vi "读取AVI文件V0（简化版）.vi"() -> ()   [LabVIEW 2013]
panel:
  in  "延时":u32
  in  "value":bool
  in  "AVI File Path":path
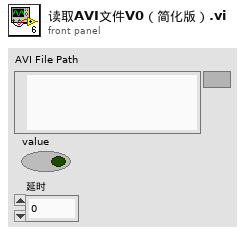
[diagram p1: front panel]
types:
  T1 = typedef "IMAQ AVI2 Refnum.ctl" = refnum<k20>
  T2 = typedef "Image Type" = u32
  T3 = typedef "IMAQ Image.ctl" = refnum<image>
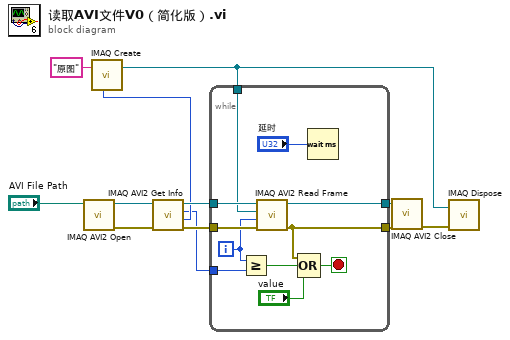
[diagram p0: block diagram]
diagram:
  n1 = call "IMAQ AVI2 Open"("AVI File Path"="AVI File Path") -> ("error out"=w11:errorcluster, "AVI Refnum"=w12:T1)  [unwired: 9 in]
  n2 = call "IMAQ AVI2 Get Info"("error in (no error)"=w11, "AVI Refnum"=w12) -> ("error out"=w10:errorcluster, "Image Type"=w8:T2, "Number of Frames"=w1:u32, "AVI Refnum (duplicate)"=w9:T1)  [unwired: 5 in, 1 out]
  n3 = call "IMAQ Create"("Image Name"="原图", "Image Type"=w8) -> ("New Image"=w2:T3)  [unwired: 3 in, 1 out]
  n4 = while {
    tunnel: w10 -> [w23]
    tunnel: w9 -> [w22]
    tunnel: w2 -> [w21]
    tunnel: [w20] -> w5
    tunnel: [w16] -> w4
    tunnel: w1 -> [w18]
    i -> [w19]
    stop <- w15 stop-if-true
    n5 = Greater Or Equal?(x=w19, y=w18) -> (x >= y?=w17:bool)
    n6 = call "IMAQ AVI2 Read Frame"("error in (no error)"=w23, "Frame Number"=w19, "Image"=w21, "AVI Refnum"=w22) -> ("error out"=w16:errorcluster, "AVI Refnum (duplicate)"=w20:T1)  [unwired: 5 in, 1 out]
    n7 = Compound Arithmetic op=OR(w16, w17, "value") -> (w15:bool)
    n8 = Wait (ms)(milliseconds to wait="延时") -> ()  [unwired: 1 out]
  }
  n9 = call "IMAQ AVI2 Close"("error in (no error)"=w4, "AVI Refnum"=w5) -> ("error out"=w3:errorcluster)  [unwired: 9 in]
  n10 = call "IMAQ Dispose"("Image"=w2, "error in (no error)"=w3) -> ()  [unwired: 4 in, 1 out]
